vi "Compute action.vi"(11 "Iteration":i32) -> (3 "Action":T1)   [LabVIEW 2010, in "XNET Reflective Memory Custom Device.lvlib"]
uses:
  XNET Reflective Memory Custom Device.lvlib
  Action.ctl
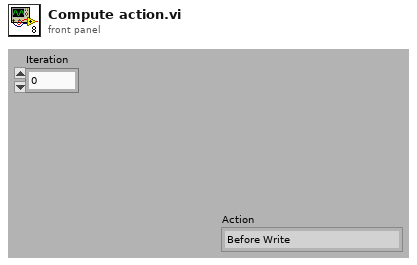
[diagram p1: front panel]
types:
  T1 = typedef "XNET Reflective Memory Custom Device.lvlib/Action.ctl" = enum16{"Before Write", "After Read", "After Write", "Before Read", "None"}
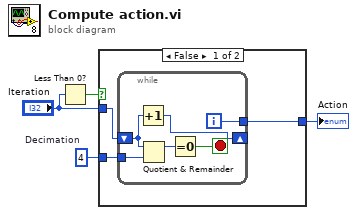
[diagram p0: block diagram]
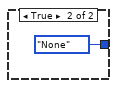
[diagram p2: hidden frame]
diagram:
  w2 = 4  # Decimation
  n1 = Less Than 0?(x="Iteration") -> (x < 0?=w4:bool)
  n2 = case shown="False" w4 {
    tunnel: [w5 Action."None" ("Action")] -> w3
    tunnel: w2 -> [w7 _]
    tunnel: "Iteration" -> [w6 _]
    frame False {
      n3 = while {
        tunnel: w7 -> [w12]
        shift-right: [w10] -> _
        shift-left: w6 -> [w9]
        tunnel: [w8] -> w5
        i -> [w8]
        stop <- w11 stop-if-true
        n4 = Increment(x=w9) -> (x+1=w10:i32)
        n5 = Quotient & Remainder(x=w9, y=w12) -> (x-y*floor(x/y)=w13:i32)  [unwired: 1 out]
        n6 = Equal To 0?(x=w13) -> (x = 0?=w11:bool)
      }
    }
    frame True {
    }
  }
  "Action" <- w3
